vi "Open and Setup CAN Session.vi"(8 "error in":errorcluster, 11 "measurement configuration":T1 {"Baudrate" format="%x"; "FD Baudrate" format="%x"}) -> (0 "error out":errorcluster, 2 "session out":refnum<k21>)   [LabVIEW 2025, in "CAN-LIN Raw Bus Capture.lvclass"]
uses:
  CAN-LIN Raw Bus Capture.lvclass
  Measurement Configuration.ctl
  CAN-LIN Raw Bus Capture UI/Toggle.ctl
  <vilib>/xnet/xnet.llb/XNET Create Session (Frame Input Stream).vi
  CAN-LIN Raw Bus Capture.lvclass/CAN-LIN Raw Bus Capture.ctl
  <resource>/objmgr/xnet.rc
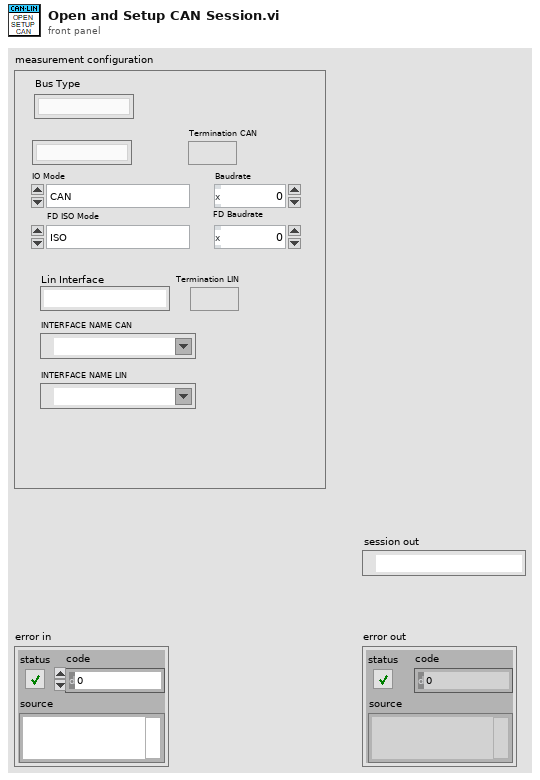
[diagram p1: front panel]
types:
  T1 = typedef "CAN-LIN Raw Bus Capture.lvclass/Measurement Configuration.ctl" = cluster{"Termination CAN":T2, "FD Baudrate":u32, "Baudrate":u32, "FD ISO Mode":enum32{"ISO", "Legacy ISO", "Non-ISO"}, "IO Mode":enum32{"CAN", "CAN FD", "CAN FD + BRS"}, "Termination LIN":T2, "Can Interface":string, "Lin Interface":string, "Bus Type":string, "INTERFACE NAME CAN":refnum<k21>, "INTERFACE NAME LIN":refnum<k21>}
  T2 = typedef "Toggle.ctl" = bool
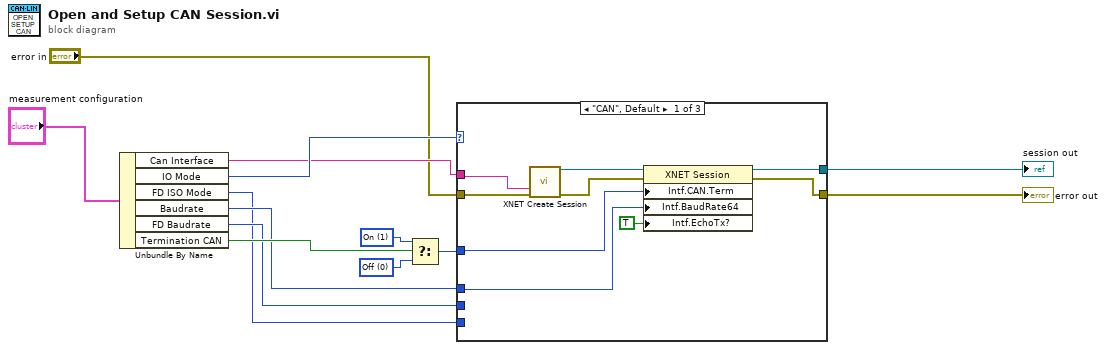
[diagram p0: block diagram]
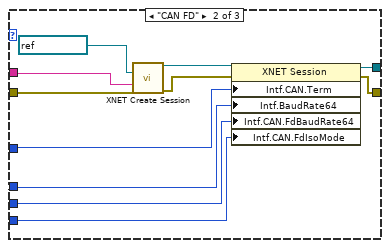
[diagram p2: hidden frame]
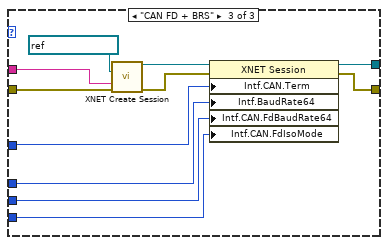
[diagram p3: hidden frame]
diagram:
  w11 = u32 1 items=["Off", "On"] ("Interface:CAN:Termination")
  w12 = u32 0 items=["Off", "On"] ("Interface:CAN:Termination")
  n1 = Unbundle By Name("measurement configuration") -> ("Can Interface"=w5:string, "IO Mode"=w10:enum32{"CAN", "CAN FD", "CAN FD + BRS"}, "FD ISO Mode"=w6:enum32{"ISO", "Legacy ISO", "Non-ISO"}, "Baudrate"=w8:u32, "FD Baudrate"=w7:u32, "Termination CAN"=w13:T2)
  n2 = Select(t=w11, s=w13, f=w12) -> (s? t:f=w9:u32)
  n3 = case shown="\"CAN\", Default" w10 {
    tunnel: [w20 w26 w41] -> w1
    tunnel: w5 -> [w17 w30 w37]
    tunnel: "error in" -> [w19 w29 w36]
    tunnel: [w18 w25 w34] -> w2
    tunnel: w8 -> [w15 w28 w40]
    tunnel: w7 -> [_ w24 w39]
    tunnel: w6 -> [_ w27 w38]
    tunnel: w9 -> [w16 w23 w35]
    frame "CAN", Default {
      n4 = call-poly <vilib>:"XNET Create Session.vi"("interface"=w17, "error in (no error)"=w19) -> ("session out"=w22:refnum<k21>, "error out"=w21:errorcluster)  [unwired: 12 in]
      n5 = property class="XNET Session"(reference=w22, error in=w21, "Intf.CAN.Term"=w16, "Intf.BaudRate64"=w15, "Intf.EchoTx?"=TRUE ("Interface:Echo Transmit?")) -> (reference out=w20:refnum<k21>, error out=w18:errorcluster)
    }
    frame "CAN FD" {
      n6 = call-poly <vilib>:"XNET Create Session.vi"("cluster (:memory:)"=refnum<k21> ":can_fd:", "interface"=w30, "error in (no error)"=w29) -> ("session out"=w32:refnum<k21>, "error out"=w31:errorcluster)  [unwired: 11 in]
      n7 = property class="XNET Session"(reference=w32, error in=w31, "Intf.CAN.Term"=w23, "Intf.BaudRate64"=w28, "Intf.CAN.FdBaudRate64"=w24, "Intf.CAN.FdIsoMode"=w27) -> (reference out=w26:refnum<k21>, error out=w25:errorcluster)
    }
    frame "CAN FD + BRS" {
      n8 = call-poly <vilib>:"XNET Create Session.vi"("cluster (:memory:)"=refnum<k21> ":can_fd_brs:", "interface"=w37, "error in (no error)"=w36) -> ("session out"=w43:refnum<k21>, "error out"=w42:errorcluster)  [unwired: 11 in]
      n9 = property class="XNET Session"(reference=w43, error in=w42, "Intf.CAN.Term"=w35, "Intf.BaudRate64"=w40, "Intf.CAN.FdBaudRate64"=w39, "Intf.CAN.FdIsoMode"=w38) -> (reference out=w41:refnum<k21>, error out=w34:errorcluster)
    }
  }
  "error out" <- w2
  "session out" <- w1
